vi "Get Image.vi"(8 "error in":errorcluster, 11 "Refnum in":refnum<k21>) -> (0 "error out":errorcluster, 2 "element":T1 {"component type" items=["standard", "hidden", "system", "unknown", "startup", "image", "essential"]}, 3 "Refnum out":refnum<k21>)   [LabVIEW 2020]
doc: "Get the most updated system image information installed in the local system."
uses:
  <vilib>/nisyscfg/Software 1.2.ctl
  <vilib>/nisyscfg/Component Type.ctl
  <vilib>/nisyscfg/Get Filtered Base System Images.vi
  <vilib>/nisyscfg/nisyscfg.lvlib
  <resource>/objmgr/nisysapi.rc
panel:
  out "Operating System:Architecture":string
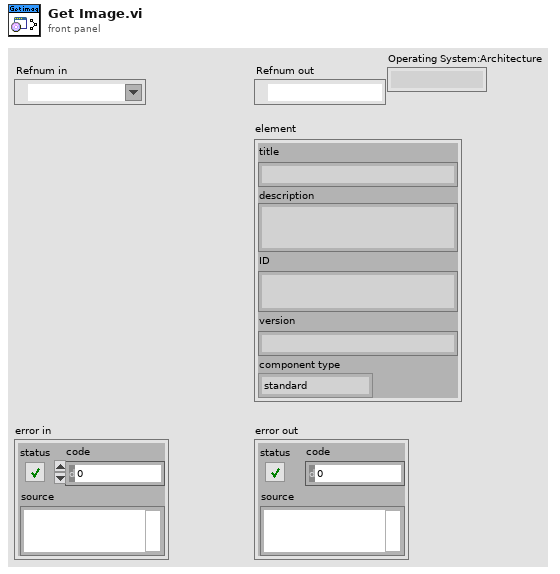
[diagram p1: front panel]
types:
  T1 = typedef "nisyscfg.lvlib/Software 1.2.ctl" = cluster{"title":string, "description":string, "ID":string, "version":string, "component type":T2}
  T2 = typedef "nisyscfg.lvlib/Component Type.ctl" = u32
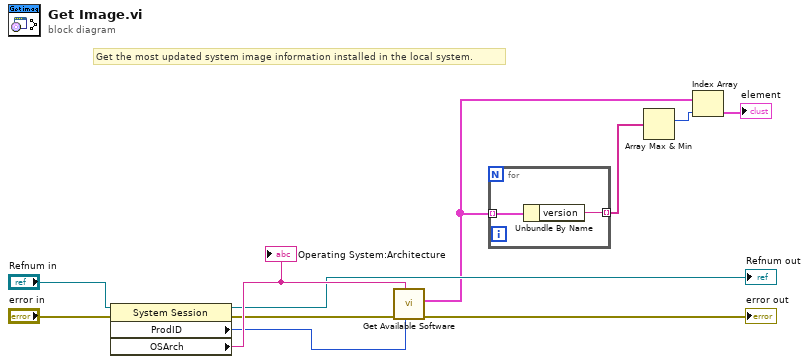
[diagram p0: block diagram]
diagram:
  # "Get the most updated system image information installed in the local system."
  n1 = property class="System Session"(reference="Refnum in", error in="error in") -> (reference out=→"Refnum out":refnum<k21>, error out=w8:errorcluster, "ProdID"=w9:i32, "OSArch"=w10:string)
  "Operating System:Architecture" <- w10
  n2 = call-poly <vilib>:"Get Available Software.vi"("Product ID"=w9, "Operating System"=w10, "error in (no error)"=w8) -> ("error out"=→"error out":errorcluster, "Base System Images"=w2:T1[])  [unwired: 6 in, 1 out]
  n3 = for {
    tunnel: w2 -> [w13] mode=indexing
    tunnel: [w12] -> w4 mode=indexing
    n4 = Unbundle By Name(w13) -> ("version"=w12:string)
  }
  n5 = Array Max & Min(array=w4) -> (max index (indices)=w3:i32)  [unwired: 3 out]
  n6 = Index Array(array=w2, index=w3) -> (element=→"element":T1)
